vi "About.vi"(8 "error in (no error)":errorcluster) -> (0 "error out":errorcluster)   [LabVIEW 2016]
doc: "Shows the about dialog"
panel:
  out "License":string
  out "Author":string="Albert Lederer, albert.d.lederer (at) googlemail.com"
  out "Version":string="16.0f2"
  out "Application Title":string="LabVIEW.exe"
  in  "OK Button":bool
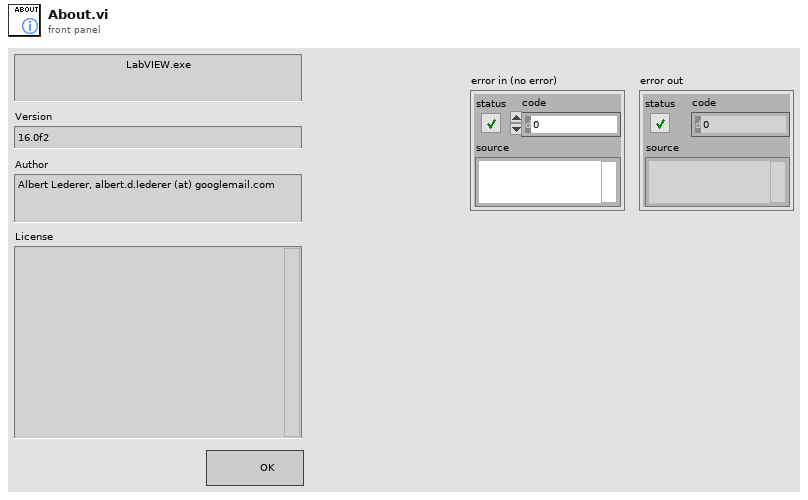
[diagram p1: front panel]
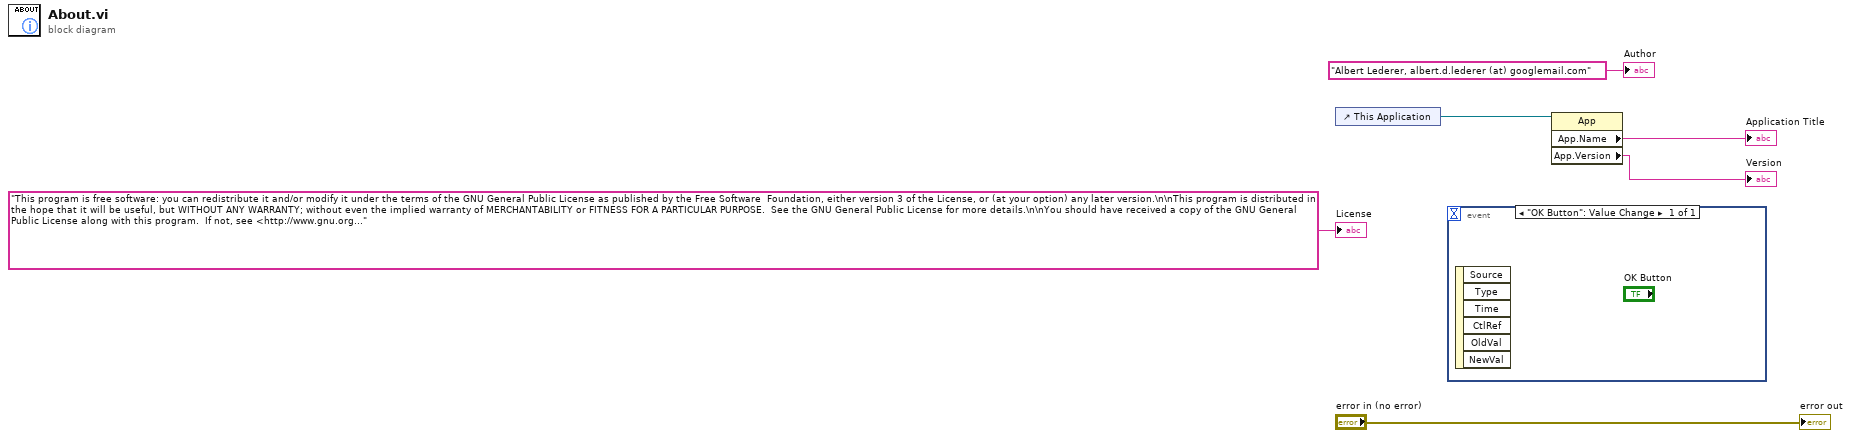
[diagram p0: block diagram]
diagram:
  n1 = control-ref of="This Application"() -> (w5:refnum<vi>)
  n2 = event shown="[0] \"OK Button\": Value Change" {
    selector: _ -> [_]
    dyn-events: _ -> [_]
    timeout: _ -> [_]
    event "OK Button": Value Change {
      n3 = event-data() -> ()  [unwired: 1 in, 6 out]
    }
  }
  n4 = property class="App"(reference=w5) -> ("App.Name"=→"Application Title":string, "App.Version"=→"Version":string)  [unwired: 1 in, 2 out]
  "error out" <- "error in (no error)"
  "Author" <- "Albert Lederer, albert.d.lederer (at) googlemail.com" ("Author")
  "License" <- "This program is free software: you can redistribute it and/or modify it under the terms of the GNU General Public License as published by the Free Software  Foundation, either version 3 of the License, or (at your option) any later version.\n\nThis program is distributed in the hope that it will be useful, but WITHOUT ANY WARRANTY; without even the implied warranty of MERCHANTABILITY or FITNESS FOR A PARTICULAR PURPOSE.  See the GNU General Public License for more details.\n\nYou should have received a copy of the GNU General Public License along with this program.  If not, see <http://www.gnu.org/licenses/>." ("License")
